vi "Resideo Read Data.vi"() -> ()   [LabVIEW 2020]
uses:
  Type Definitions/Vesta Info.ctl
panel:
  out "Vesta Data Output":T1
  in  "stop":bool
  out "error out":errorcluster
  in  "error in (no error)":errorcluster
  in  "VISA resource name":refnum<visa-resource-name>
  in  "Use Vesta Tool?":bool
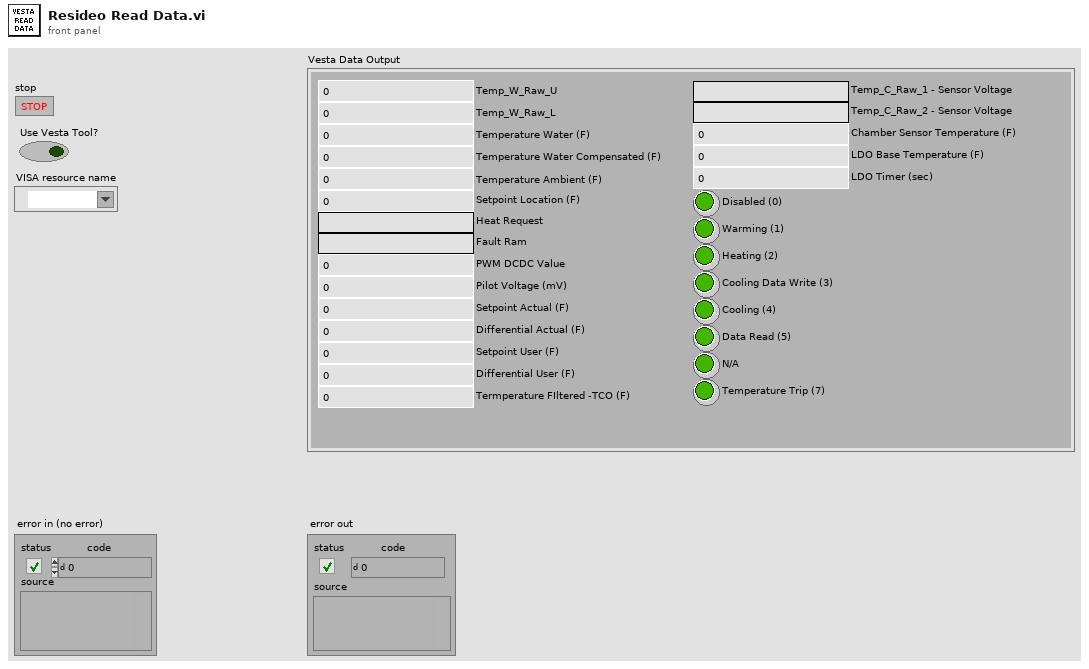
[diagram p1: front panel]
types:
  T1 = typedef "Vesta Info.ctl" = cluster{"Temp_W_Raw_U":u16, "Temp_W_Raw_L":u16, "Temperature Water (F)":dbl, "Temperature Water Compensated (F)":dbl, "Temperature Ambient (F)":dbl, "Setpoint Location (F)":dbl, "Heat Request":string, "Fault Ram":string, "PWM DCDC Value":u16, "Pilot Voltage (mV)":dbl, "Setpoint Actual (F)":dbl, "Differential Actual (F)":dbl, "Setpoint User (F)":dbl, "Differential User (F)":dbl, "Termperature FIltered -TCO (F)":dbl, "Temp_C_Raw_1 - Sensor Voltage":string, "Temp_C_Raw_2 - Sensor Voltage":string, "Chamber Sensor Temperature (F)":dbl, "LDO Base Temperature (F)":dbl, "LDO Timer (sec)":i16, "Disabled (0)":bool, "Warming (1)":bool, "Heating (2)":bool, "Cooling Data Write (3)":bool, "Cooling (4)":bool, "Data Read (5)":bool, "N/A":bool, "Temperature Trip (7)":bool}
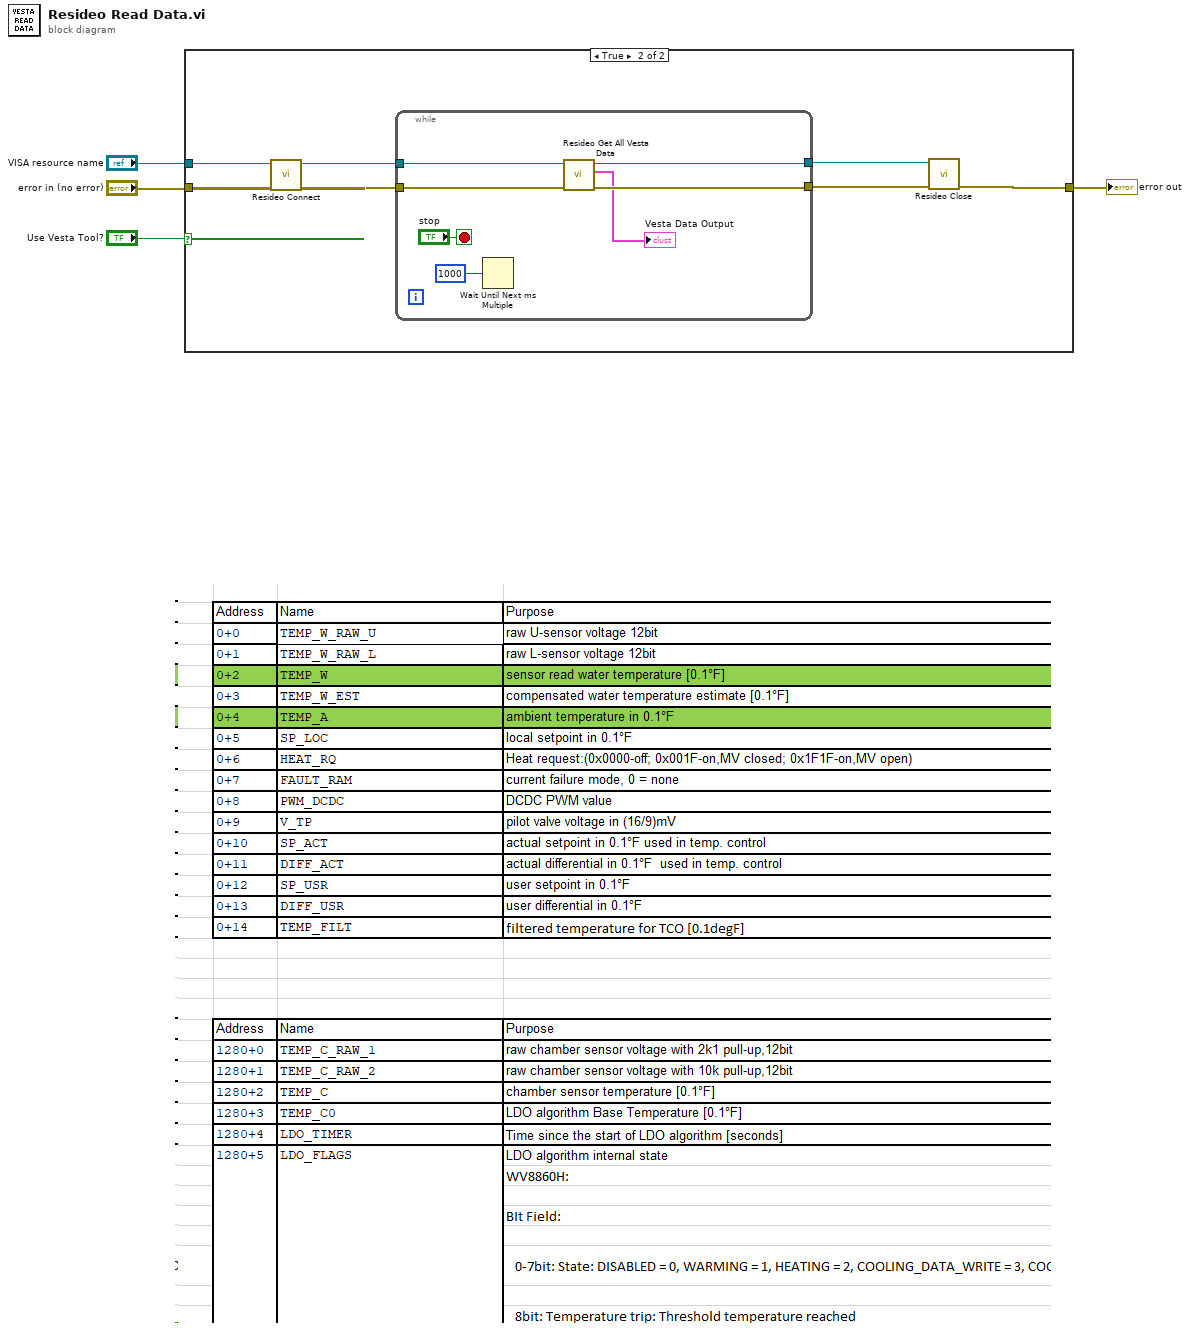
[diagram p0: block diagram]
diagram:
  n1 = case shown="True" "Use Vesta Tool?" {
    tunnel: "VISA resource name" -> [_ w12]
    tunnel: "error in (no error)" -> [w5 w11]
    tunnel: [w5 w10] -> w2
    frame False {
    }
    frame True {
      n2 = call "Resideo Connect.vi"("error in (no error)"=w11, "VISA Refnum in"=w12) -> ("error out"=w9:errorcluster, "Modbus Master out"=w8:refnum<class "Modbus Master.lvclass">)  [unwired: 8 in]
      n3 = while {
        tunnel: w9 -> [w17]
        tunnel: w8 -> [w18]
        tunnel: [w14] -> w7
        tunnel: [w15] -> w6
        stop <- "stop" stop-if-true
        n4 = Wait Until Next ms Multiple(millisecond multiple=u32 1000) -> ()  [unwired: 1 out]
        n5 = call "Resideo Get All Vesta Data.vi"("error in (no error)"=w17, "Modbus Master in"=w18) -> ("error out"=w14:errorcluster, "Vesta Data Output"=→"Vesta Data Output":T1, "Modbus Master out"=w15:refnum<class "Modbus Master.lvclass">)  [unwired: 7 in]
      }
      n6 = call "Resideo Close.vi"("error in (no error)"=w7, "Modbus Master in"=w6) -> ("error out"=w10:errorcluster)  [unwired: 9 in]
    }
  }
  "error out" <- w2
